vi "PH_BlackBox.set i Attr.vi"(0 "VI in":refnum<vi>, 5 "error in (no error)":errorcluster) -> (14 "VI out":refnum<vi>, 16 "i Attribute":T1 {"Position OUT" items=["no info", "off/false/out", "on/true/in", "Failure", "Alarm", "Status 1", "Status 2", "Status 3"]; "Position IN" items=["no info", "off/false/out", "on/true/in", "Failure", "Alarm", "Status 1", "Status 2", "Status 3"]}, 19 "error out":errorcluster)   [LabVIEW 2014, in "PH_BlackBox.lvlib"]
uses:
  PH_BlackBox.lvlib
  PH_BlackBox.i attribute.ctl
  PH_BlackBox.GUI Refs.ctl
  PH_Basics/PH_StatusHandler/PH_StatusHandler.Status.ctl
  CS_Core/CSSystem/CSSystemLib/CSSystemLib.lvlib
  PH_Basics/PH_StatusHandler/PH_StatusHandler.lvlib
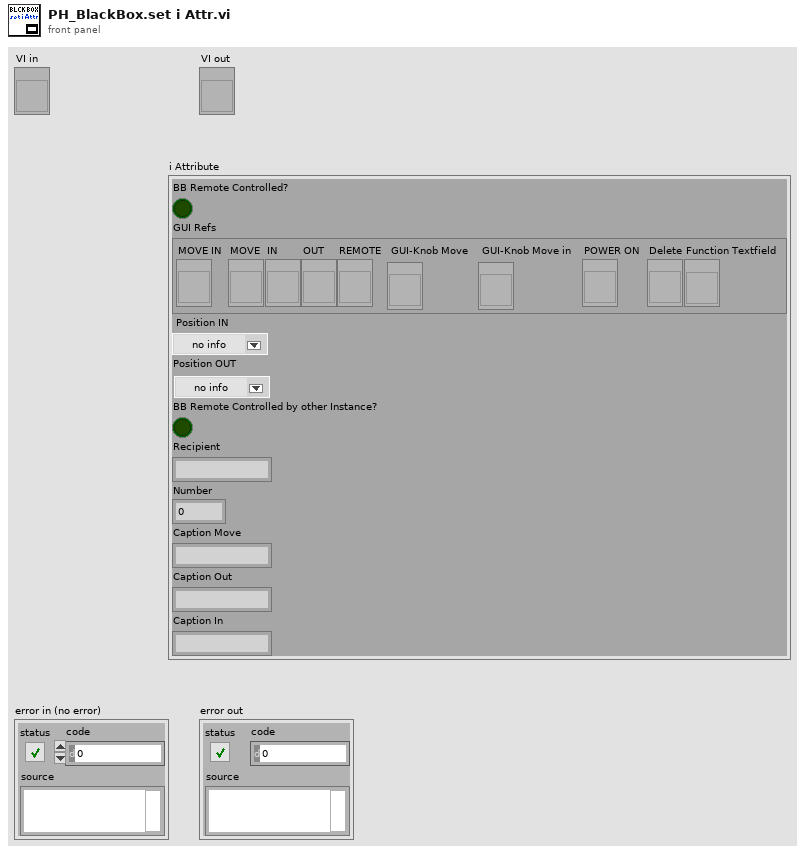
[diagram p1: front panel]
types:
  T1 = typedef "PH_BlackBox.lvlib/PH_BlackBox.i attribute.ctl" = cluster{"BB Remote Controlled?":bool, "GUI Refs":T2, "Position IN":T3, "Position OUT":T3, "BB Remote Controlled by other Instance?":bool, "Recipient":string, "Number":i32, "Caption Move":string, "Caption Out":string, "Caption In":string}
  T2 = typedef "PH_BlackBox.lvlib/PH_BlackBox.GUI Refs.ctl" = cluster{"MOVE IN":refnum<vi>, "MOVE":refnum<vi>, "IN":refnum<vi>, "OUT":refnum<vi>, "REMOTE":refnum<vi>, "GUI-Knob Move":refnum<vi>, "GUI-Knob Move in":refnum<vi>, "POWER ON":refnum<vi>, "Delete":refnum<vi>, "Function Textfield":refnum<vi>}
  T3 = typedef "PH_StatusHandler.lvlib/PH_StatusHandler.Status.ctl" = i16
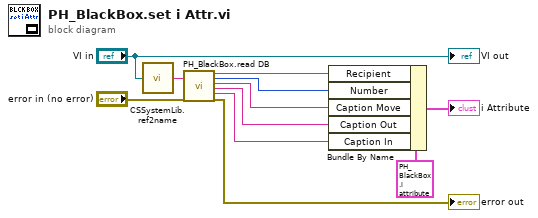
[diagram p0: block diagram]
diagram:
  n1 = call "CSSystemLib.ref2name.vi"("obj refnum"="VI in") -> ("name"=w8:string)
  n2 = call "PH_BlackBox.read DB.vi"("BB Instance"=w8, "error in (no error)"="error in (no error)") -> ("Recipient"=w7:string, "#"=w3:i32, "Caption Move"=w6:string, "Caption Out"=w5:string, "Caption In"=w4:string, "error out"=→"error out":errorcluster)  [unwired: 12 in]
  n3 = Bundle By Name(cluster=T1 {"BB Remote Controlled?"=FALSE, "GUI Refs"={"MOVE IN"=refnum, "MOVE"=refnum, "IN"=refnum, "OUT"=refnum, "REMOTE"=refnum, "GUI-Knob Move"=refnum, "GUI-Knob Move in"=refnum, "POWER ON"=refnum, "Delete"=refnum, "Function Textfield"=refnum}, "Position IN"=0, "Position OUT"=0, "BB Remote Controlled by other Instance?"=FALSE, "Recipient"="N/A", "Number"=0, "Caption Move"="", "Caption Out"="", "Caption In"=""} ("CLASS.i attribute"), "Recipient"=w7, "Number"=w3, "Caption Move"=w6, "Caption Out"=w5, "Caption In"=w4) -> (→"i Attribute":T1)
  "VI out" <- "VI in"
